vi "OFBS_shuffleTrainingData.vi"(8 "error in (no error)":errorcluster, 11 "OptFreqBandsSearch in":refnum<class "OptFreqBandsSearch.lvclass">) -> (0 "error out":errorcluster, 3 "OptFreqBandsSearch out":refnum<class "OptFreqBandsSearch.lvclass">)   [LabVIEW 2016, in "Optimal Frequency Bands Search.lvlib" / "OptFreqBandsSearch.lvclass"]
uses:
  OptFreqBandsSearch.lvclass
  OptFreqBandsSearch.lvclass/OptFreqBandsSearch.ctl
  Optimal Frequency Bands Search.lvlib
panel:
  # "This VI is a part of BCI Design library, http://www.ru-bci.org \nCopyright © 2020, Sotnikov Peter, All rights reserved. License: CC BY-NC 4.0"
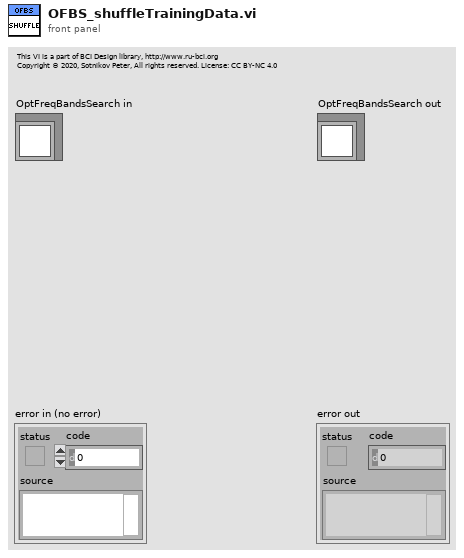
[diagram p1: front panel]
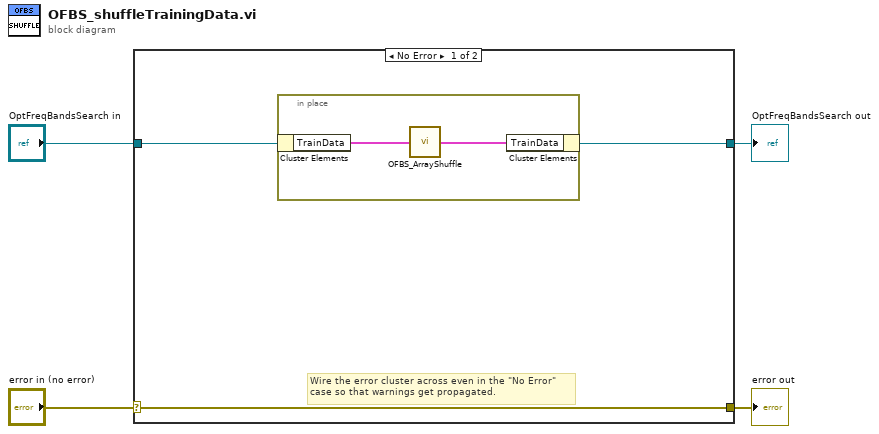
[diagram p0: block diagram]
diagram:
  n1 = case shown="No Error" "error in (no error)" {
    selector: "error in (no error)" -> [w7 w11]
    tunnel: [w7 w11] -> w3
    tunnel: [w5 w10] -> w1
    tunnel: "OptFreqBandsSearch in" -> [w6 w10]
    frame No Error {
      # "Wire the error cluster across even in the \"No Error\"\ncase so that warnings get propagated."
      n2 = in-place {
        n3 = in-place-cluster #1(w6) -> ("TrainData"=w9:cluster{"ClassLabel":string, "Trial":dbl[][]}[])
        n4 = call "OFBS_ArrayShuffle.vi"("Array in"=w9) -> ("Array out"=w8:cluster{"ClassLabel":string, "Trial":dbl[][]}[])
        n5 = in-place-cluster #1("TrainData"=w8) -> (w5:refnum<class "OptFreqBandsSearch.lvclass">)
      }
    }
    frame Error {
    }
  }
  "error out" <- w3
  "OptFreqBandsSearch out" <- w1
